vi "Set Time Stamp.vi"(8 "error in (no error)":errorcluster, 10 "Time Stamp":timestamp, 11 "Record in":refnum<class "Record.lvclass">) -> (0 "error out":errorcluster, 3 "Record out":refnum<class "Record.lvclass">)   [LabVIEW 2017, in "Error Log.lvlib" / "Record.lvclass"]
uses:
  Record.lvclass
  Record.lvclass/Record.ctl
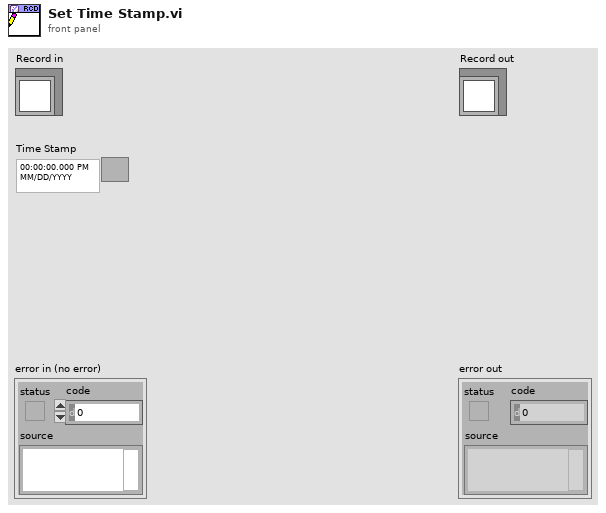
[diagram p1: front panel]
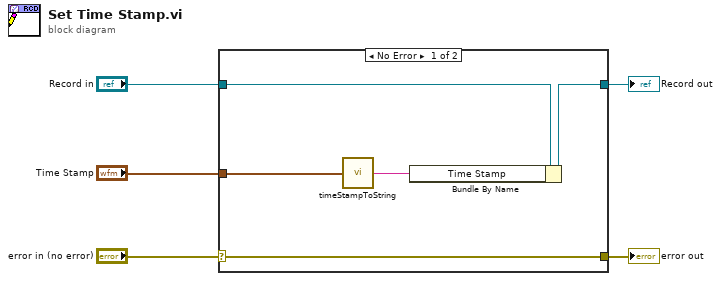
[diagram p0: block diagram]
diagram:
  n1 = case shown="No Error" "error in (no error)" {
    selector: "error in (no error)" -> [w10 w11]
    tunnel: [w10 w11] -> w4
    tunnel: [w8 w12] -> w2
    tunnel: "Record in" -> [w9 w12]
    tunnel: "Time Stamp" -> [w7 _]
    frame No Error {
      n2 = call "timeStampToString.vi"("Time Stamp"=w7) -> ("Time Stamp String"=w6:string)
      n3 = Bundle By Name(cluster=w9, "Time Stamp"=w6) -> (w8:refnum<class "Record.lvclass">)
    }
    frame Error {
    }
  }
  "error out" <- w4
  "Record out" <- w2
